vi "chart color.vi"(8 "错误输入（无错误）":errorcluster caption="error in", 11 "Chart ref in":refnum<vi>) -> (0 "错误输出":errorcluster caption="error out", 3 "Chart ref out":refnum<vi>)   [LabVIEW 2011]
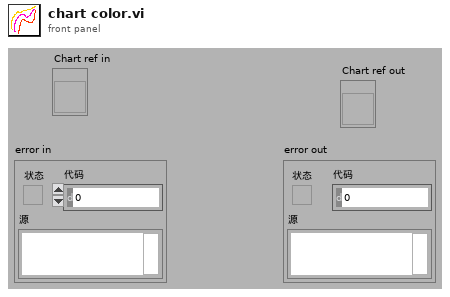
[diagram p1: front panel]
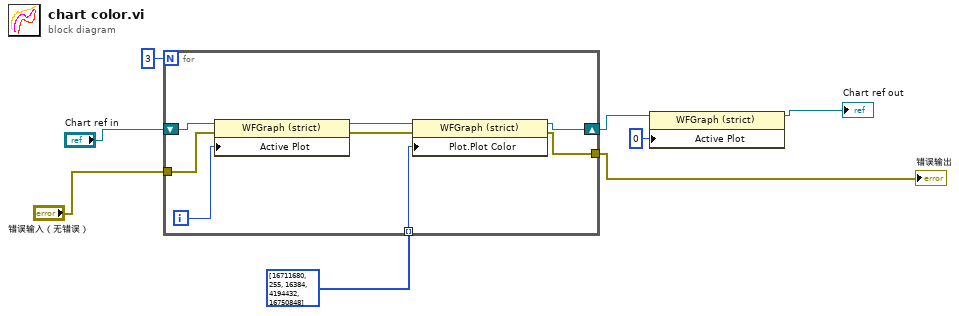
[diagram p0: block diagram]
diagram:
  n1 = for {
    N: 3 -> [_]
    tunnel: u32[] [16711680, 255, 16384, 4194432, 16750848] -> [w12] mode=indexing
    tunnel: "错误输入（无错误）" -> [w10]
    tunnel: [w9] -> w4
    shift-right: [w13] -> w3
    shift-left: "Chart ref in" -> [w16]
    i -> [w15]
    n2 = property class="WFGraph (strict)"(reference=w16, error in=w10, "Active Plot"=w15) -> (reference out=w14:refnum<vi>, error out=w11:errorcluster)
    n3 = property class="WFGraph (strict)"(reference=w14, error in=w11, "Plot.Plot Color"=w12) -> (reference out=w13:refnum<vi>, error out=w9:errorcluster)
  }
  "错误输出" <- w4
  n4 = property class="WFGraph (strict)"(reference=w3, "Active Plot"=u32 0 ("活动曲线")) -> (reference out=→"Chart ref out":refnum<vi>)  [unwired: 1 in, 1 out]
